vi "UI.vi"() -> ()   [LabVIEW 2015]
panel:
  in  "stop":bool
  in  "Last Update":dbl
  out "_timestamp":timestamp caption="Last Update" format="%<%I:%M:%S %p\n%x>T"
  out "U8_input":u8 caption="U8"
  out "U16_input":u16 caption="U16"
  out "U32_input":u32 caption="U32"
  out "U64_input":u64 caption="U64"
  out "I8_input":i8 caption="I8"
  out "I16_input":i16 caption="I16"
  out "I32_input":i32 caption="I32"
  out "I64_input":i64 caption="I64"
  out "Single_input":sgl caption="Single"
  out "Double_input":dbl caption="Double"
  out "Boolean_input":bool caption="Boolean"
  in  "U8_output":u8 caption="U8"
  in  "U16_output":u16 caption="U16"
  in  "U32_output":u32 caption="U32"
  in  "U64_output":u64 caption="U64"
  in  "I8_output":i8 caption="I8"
  in  "I16_output":i16 caption="I16"
  in  "I32_output":i32 caption="I32"
  in  "I64_output":i64 caption="I64"
  in  "Single_output":sgl caption="Single"
  in  "Double_output":dbl caption="Double"
  in  "Boolean_output":bool caption="Boolean"
  # "Inputs"
  # "Outputs"
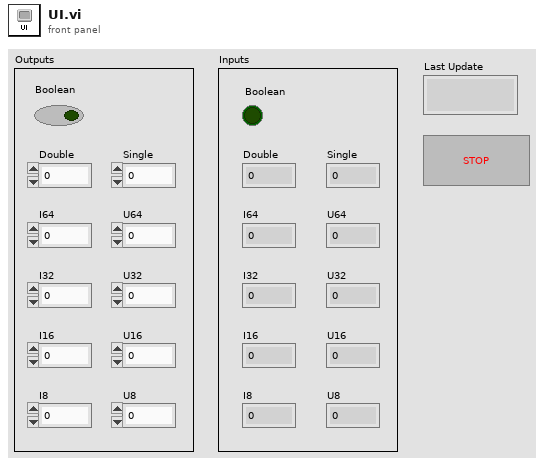
[diagram p1: front panel]
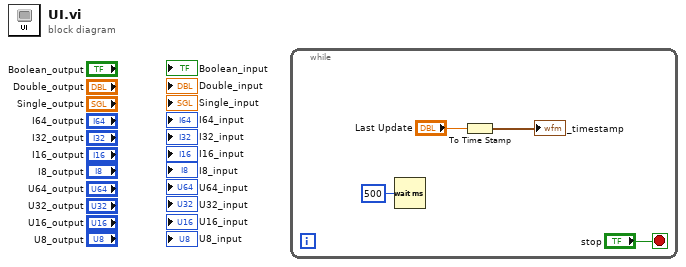
[diagram p0: block diagram]
diagram:
  n1 = while {
    stop <- "stop" stop-if-true
    n2 = Wait (ms)(milliseconds to wait=u32 500) -> ()  [unwired: 1 out]
    n3 = To Time Stamp(1:"Last Update") -> (0:→"_timestamp":timestamp)
  }
